vi "Sending_Seek_Recipe_Sub_VI.vi"(0 "connection ID":refnum<k5>, 3 "Receipe Msg ID":i32, 4 "Receipe Message length":i32, 5 "SeekTime":i32, 6 "MemoryClearBeforeSeek":i32, 7 "SeekAmplitudeLoopC1":i32, 8 "SeekAmplitudeLoopC2":i32, 9 "SeekFreqLimitHigh":i32, 10 "SeekPhaseloopCF":i32, 12 "SeekFreqLimitLow":i32, 13 "SeekPhaseloopI":i32, 15 "SeekRampTime":i32, 16 "SeekFreqOffset":i32, 17 "error input":errorcluster, 20 "Response ID":u8=66) -> (21 "connection ID":refnum<k5>, 24 "error out":errorcluster)   [LabVIEW 2017]
panel:
  out "rest of the binary string":string
  out "*(type *) &x 2":u8
  out "*(type *) &x":u8
  out "String":string=" Success"
  out "bytes written":i32
  # "For 20 KHZ\n                                  INT32 SeekTime = 500\n                                  INT32 SeekAmplitudeLoopC1 = 205\n                                  INT32 SeekAmplitudeLoopC2 =  370\n                                  INT32 SeekFreqLimitHigh = 410000\n                                  INT32 SeekFreqLimitLow = 390000\n                                  INT32 SeekPhaseloopI = 140\n                                  INT32 SeekPhaseloopCF = 200\n                                  INT32 SeekRampTime =  500\n                                  INT32 SeekFreqOffset=  0"
  # "Please find the below information,\n                               \n                                                                Default                 Min                        Max\n \nSeekTime                                            500ms                   500ms                   1000ms (Note : To cross check sonic overload , It may extend up to 4000ms. But, In actual case \n                                                                                                                            1000ms(as per Girish input))\n \n20KHz System:\n-------------------\nSeekFreqLimitLow                           195000                  195000                     -\nSeekFreqLimitHigh                          205000                       -                         205000\n \n30KHz System:\n-------------------\nSeekFreqLimitLow                           292500                  292500                     -\nSeekFreqLimitHigh                          307500                       -                         307500\n \n40KHz System:\n-------------------\nSeekFreqLimitLow                           395000                  390000                     -\nSeekFreqLimitHigh                          405000                       -                         410000"
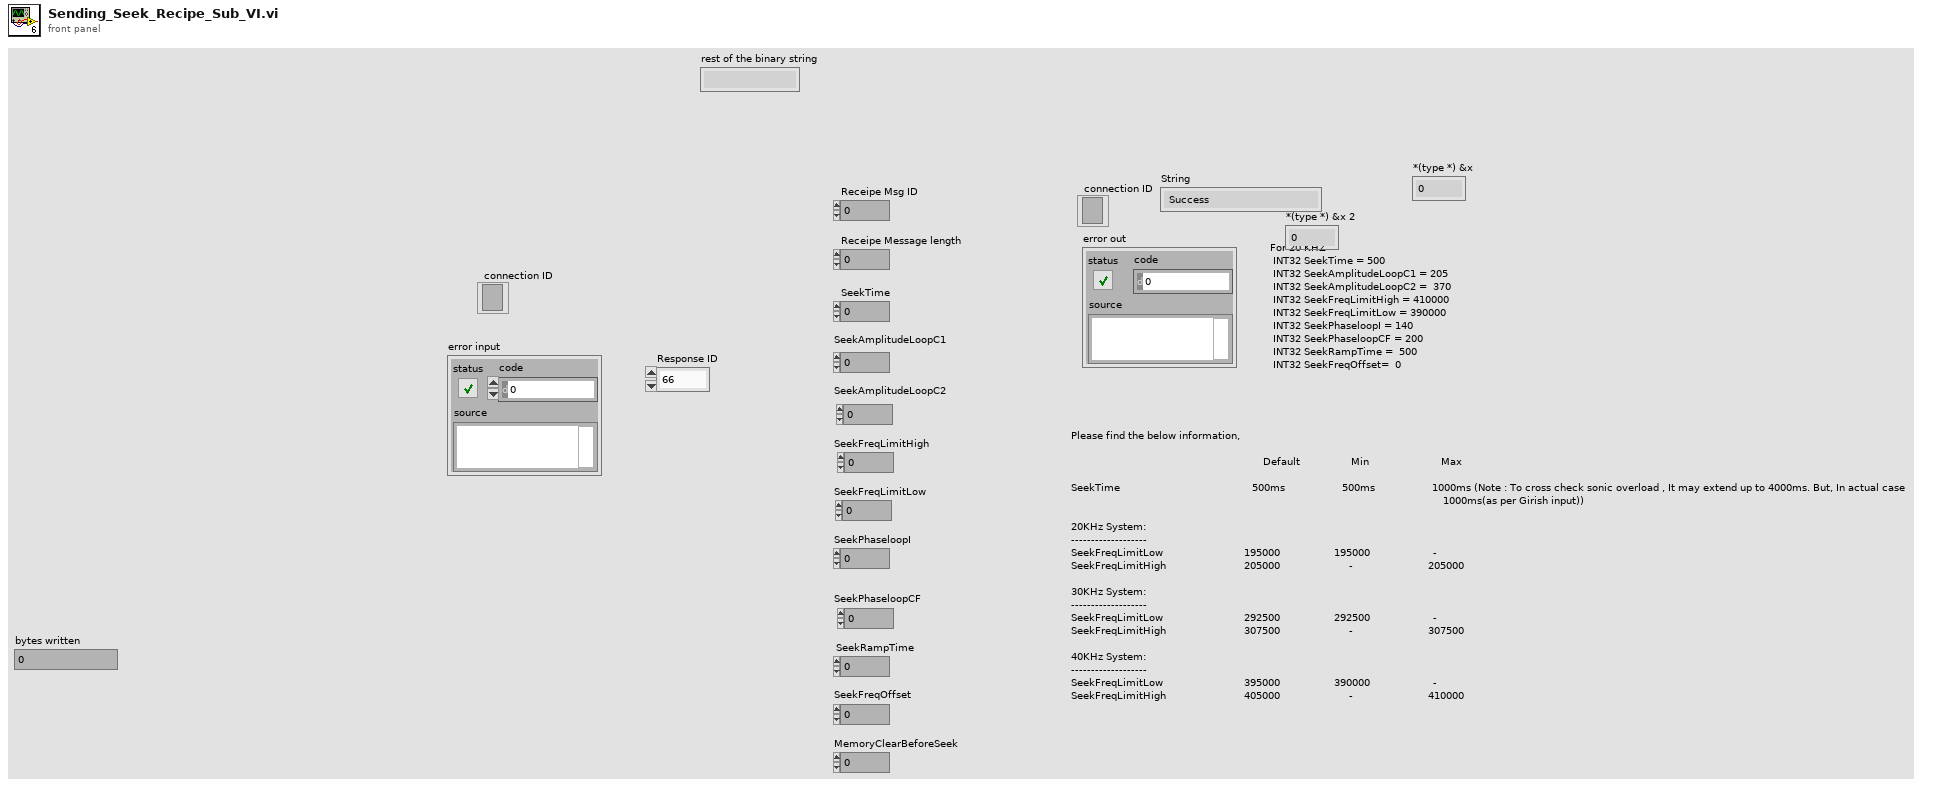
[diagram p1: front panel]
types:
  T1 = enum16{"big-endian, network order", "native, host order", "little-endian"}
  T2 = cluster{"SeekTime":i32, "MemoryClearBeforeSeek":i32, "SeekFreqOffset":i32, "SeekRampTime":i32, "SeekPhaseloopCF":i32, "SeekPhaseloopI":i32, "SeekFreqLimitLow":i32, "SeekFreqLimitHigh":i32, "SeekAmplitudeLoopC2":i32, "SeekAmplitudeLoopC1":i32, "Receipe Message length":i32, "Receipe Msg ID":i32}
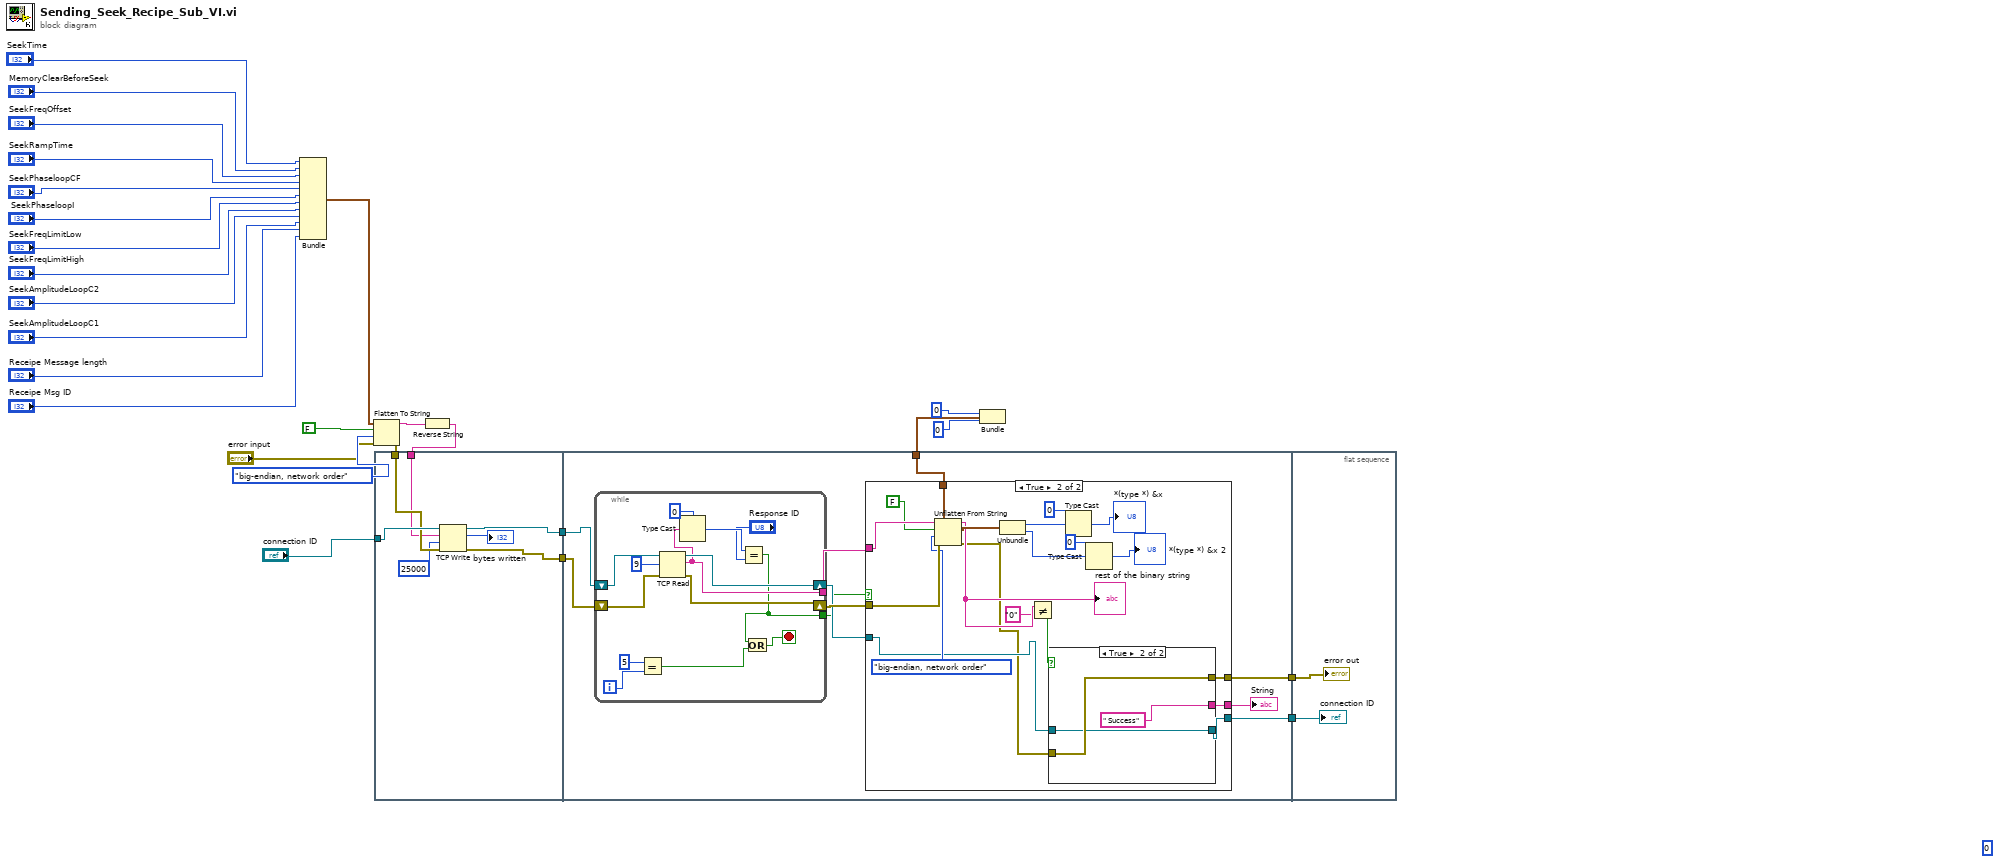
[diagram p0: block diagram]
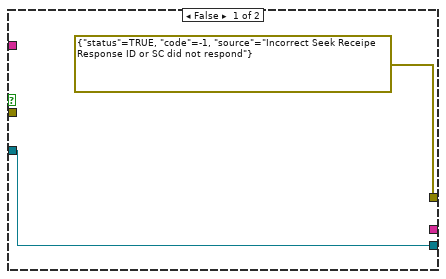
[diagram p2: hidden frame]
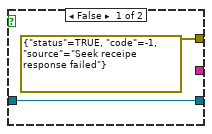
[diagram p3: hidden frame]
diagram:
  (unwired) u8 0
  n1 = Bundle("SeekTime"="SeekTime", "MemoryClearBeforeSeek"="MemoryClearBeforeSeek", "SeekFreqOffset"="SeekFreqOffset", "SeekRampTime"="SeekRampTime", "SeekPhaseloopCF"="SeekPhaseloopCF", "SeekPhaseloopI"="SeekPhaseloopI", "SeekFreqLimitLow"="SeekFreqLimitLow", "SeekFreqLimitHigh"="SeekFreqLimitHigh", "SeekAmplitudeLoopC2"="SeekAmplitudeLoopC2", "SeekAmplitudeLoopC1"="SeekAmplitudeLoopC1", "Receipe Message length"="Receipe Message length", "Receipe Msg ID"="Receipe Msg ID") -> (w20:T2)  [unwired: 1 in]
  n2 = Flatten To String(anything=w20, prepend array or string size? (T)=FALSE, byte order (0:big-endian, network order)=T1."big-endian, network order", error in (no error)="error input") -> (data string=w24:string, error out=w25:errorcluster)  [unwired: 1 out]
  n3 = flat-sequence {
    tunnel: "connection ID" -> [w34]
    tunnel: w25 -> [w33]
    tunnel: w23 -> [w32]
    tunnel: [w29] -> w12
    tunnel: [w28] -> w11
    tunnel: w17 -> [w40]
    tunnel: [w39] -> w16
    tunnel: [w38] -> w15
    tunnel: w12 -> [w36]
    tunnel: w11 -> [w35]
    tunnel: w16 -> [w87]
    tunnel: w15 -> [w86]
    frame #0 {
      n4 = TCP Write(connection ID=w34, data in=w32, error in (no error)=w33, 9:25000 ("timeout ms (25000)")) -> (connection ID out=w29:refnum<k5>, bytes written=→"bytes written":i32, error out=w28:errorcluster)
    }
    frame #1 {
      n5 = while {
        tunnel: [w81] -> w43
        shift-right: [w83] -> w42
        shift-left: w36 -> [w85]
        shift-right: [w77] -> w44
        shift-left: w35 -> [w84]
        tunnel: [w75] -> w41
        i -> [w74]
        stop <- w76 stop-if-true
        n6 = Equal?(x=5, y=w74) -> (x = y?=w72:bool)
        n7 = TCP Read(connection ID=w85, bytes to read=9, error in (no error)=w84) -> (connection ID out=w83:refnum<k5>, data out=w81:string, error out=w77:errorcluster)  [unwired: 2 in]
        n8 = Type Cast(type=u8 0, x=w81) -> (*(type *) &x=w79:u8)
        n9 = Equal?(x=w79, y="Response ID") -> (x = y?=w75:bool)
        n10 = Or(x=w75, y=w72) -> (x .or. y?=w76:bool)
      }
      n11 = case shown="True" w41 {
        tunnel: w44 -> [_ w66]
        tunnel: w43 -> [_ w65]
        tunnel: w42 -> [w46 w57]
        tunnel: w40 -> [_ w61]
        tunnel: [w46 w56] -> w39
        tunnel: [errorcluster {"status"=TRUE, "code"=-1, "source"="Incorrect Seek Receipe Response ID or SC did not respond"} ("error constant") w55] -> w38
        tunnel: [_ w54] -> w37
        frame False {
        }
        frame True {
          n12 = Unflatten From String(type=w61, binary string=w65, data includes array or string size? (T)=FALSE, byte order (0:big-endian, network order)=T1."big-endian, network order", error in (no error)=w66) -> (rest of the binary string=w60:string, value=w62:cluster{i32, i32}, error out=w53:errorcluster)
          "rest of the binary string" <- w60
          n13 = Unbundle(w62) -> (w52:i32, w47:i32)
          n14 = Not Equal?(x=w60, y="0") -> (x != y?=w58:bool)
          n15 = case shown="True" w58 {
            tunnel: [errorcluster {"status"=TRUE, "code"=-1, "source"="Seek receipe response failed"} ("error constant") w70] -> w55
            tunnel: w57 -> [w67 w69]
            tunnel: [w67 w69] -> w56
            tunnel: [_ " Success"] -> w54
            tunnel: w53 -> [_ w70]
            frame False {
            }
            frame True {
            }
          }
          n16 = Type Cast(type=u8 0, x=w52) -> (*(type *) &x=→"*(type *) &x":u8)
          n17 = Type Cast(type=u8 0, x=w47) -> (*(type *) &x=→"*(type *) &x 2":u8)
        }
      }
      "String" <- w37
    }
    frame #2 {
      "connection ID" <- w87
      "error out" <- w86
    }
  }
  n18 = Reverse String(1:w24) -> (0:w23:string)
  n19 = Bundle(0, 0) -> (w17:cluster{i32, i32})  [unwired: 1 in]
